vi "Test HS256.vi"() -> ()   [LabVIEW 2020]
uses:
  Crypto/Signatures/HMAC/HMAC.lvclass
  Crypto/Hashes/SHA-256/SHA-256.lvclass
panel:
  in  "Message":string
  out "Signature":string
  in  "Key":string
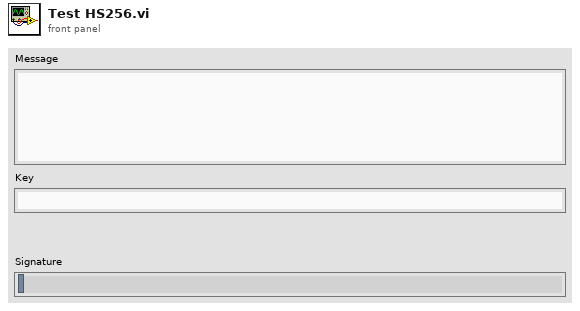
[diagram p1: front panel]
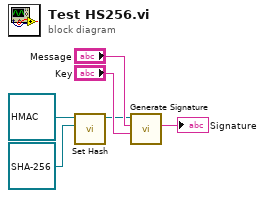
[diagram p0: block diagram]
diagram:
  n1 = call "Set Hash.vi"("Hash"=refnum<class "SHA-256.lvclass"> refnum ("Crypto.lvlib:SHA-256.lvclass"), "HMAC in"=refnum<class "HMAC.lvclass"> refnum ("Crypto.lvlib:HMAC.lvclass")) -> ("HMAC out"=w1:refnum<class "HMAC.lvclass">)  [unwired: 8 in, 1 out]
  n2 = call-dynamic "Generate Signature.vi"("Key"="Key", "Message"="Message", "HMAC in"=w1) -> ("Signature"=→"Signature":string)  [unwired: 6 in, 2 out]
